vi "parseAddress.vi"(8 "error in (no error)":errorcluster, 11 "FrameParser in":refnum<class "DynamicFrameParser.lvclass">) -> (0 "error out":errorcluster, 2 "Address":u8, 3 "FrameParser out":refnum<class "DynamicFrameParser.lvclass">)   [LabVIEW 2016, in "RTModbus.lvlib" / "DynamicFrameParser.lvclass"]
uses:
  DynamicFrameParser.lvclass
  DynamicFrameParser.lvclass/DynamicFrameParser.ctl
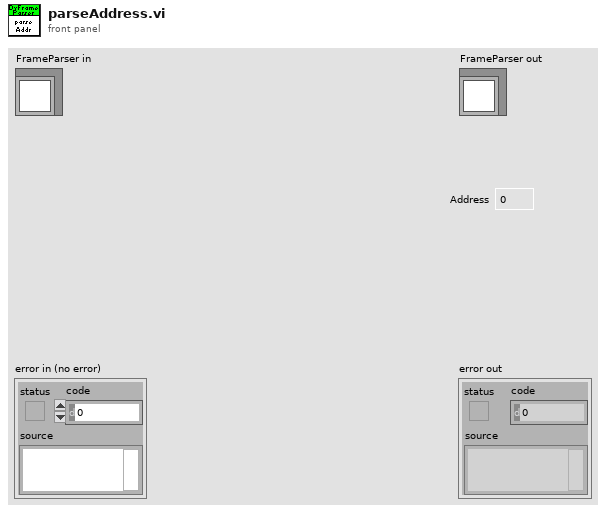
[diagram p1: front panel]
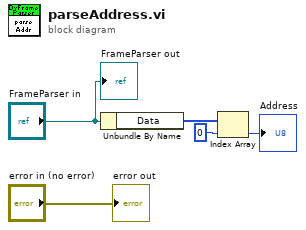
[diagram p0: block diagram]
diagram:
  n1 = Unbundle By Name("FrameParser in") -> ("Data"=w5:u8[])
  n2 = Index Array(array=w5, index=0) -> (element=→"Address":u8)
  "error out" <- "error in (no error)"
  "FrameParser out" <- "FrameParser in"
